vi "Teleop.vi"(1 "PreValue 2":bool, 3 "PreValue":bool, 9 "PreValue 3":bool, 10 "Match Info":T1={"Autonomous Elapsed Seconds"=0.0, "TeleOp Elapsed Seconds"=0.0, "Disabled Elapsed Seconds"=0.0, "Visited Autonomous"=FALSE, "Visited TeleOp"=FALSE, "Visited Disabled"=FALSE, "Autonomous Settings"={"Autonomous Style"=enum."Independent", "VI Refnum"=refnum}}, 11 "Call Context":T2) -> (0 "CurrentValue 2":bool, 2 "CurrentValue":bool, 8 "CurrentValue 3":bool)   [LabVIEW 2015]
doc: "This VI is called for each TeleOp packet received from the DS where the robot is not disabled. It is often used to read from the joysticks and update I/O or to update setpoints for timed control loops. It should complete and return within 20 milliseconds or it may miss DS packets."
uses:
  <vilib>/Rock Robotics/WPI/DriverStation/WPI_DriverStationDerivedRobotMode.ctl
  <vilib>/Rock Robotics/WPI/DriverStation/WPI_DriverStationMatch Info.ctl
  <vilib>/Rock Robotics/WPI/Solenoid/WPI_SolenoidValue.ctl
  <vilib>/Rock Robotics/WPI/Utilities/WPI_GetSetVariantRefNum.vi
  <vilib>/Rock Robotics/Network Tables/NT Write Boolean.vi
  <vilib>/Rock Robotics/Network Tables/NT Write Numeric Array.vi
  <vilib>/Rock Robotics/Network Tables/NT Read Boolean.vi
  <vilib>/Rock Robotics/Network Tables/NT Read Number.vi
  Robot Global Data.vi
  <vilib>/Rock Robotics/WPI/Solenoid/WPI_SolenoidSetEnum.vi
panel:
  out "Sample Slider 0":dbl(slide) scale=0.0..5.0
  out "Sample Boolean 1":bool
  out "Sample Boolean 0":bool
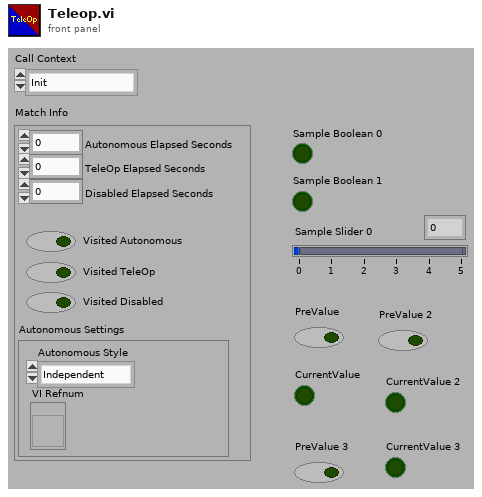
[diagram p1: front panel]
types:
  T1 = typedef "WPI_DriverStationMatch Info.ctl" = cluster{"Autonomous Elapsed Seconds":dbl, "TeleOp Elapsed Seconds":dbl, "Disabled Elapsed Seconds":dbl, "Visited Autonomous":bool, "Visited TeleOp":bool, "Visited Disabled":bool, "Autonomous Settings":cluster{"Autonomous Style":enum16{"Iterative", "Independent"}, "VI Refnum":refnum<vi>}}
  T2 = typedef "WPI_DriverStationDerivedRobotMode.ctl" = enum16{"Init", "Execute", "Stop"}
  T3 = typedef "WPI_RobotDriveDevRef.ctl" = cluster{"DevStatus":errorcluster, "Motors[]":T4[], "Square Inputs":bool, "Max Output":dbl}
  T4 = typedef "WPI_MotorControlDeviceRef.ctl" = cluster{"DeviceStatus":errorcluster, "Type":T5, "PWM":cluster{"PWM Channel":T6, "DeadBand":T7}, "CAN":cluster{"Device Number":u8, "Control Mode":T8, "Semaphore":T9, "Max Vout":dbl, "TalonSRX Control Mode":T10}, "Invert":bool}
  T5 = typedef "WPI_MotorControlType.ctl" = enum16{"PWM", "CAN", "CANTalonSRX"}
  T6 = typedef "FPGA_DIOPWMChannel.ctl" = enum8{"PWM 0", "PWM 1", "PWM 2", "PWM 3", "PWM 4", "PWM 5", "PWM 6", "PWM 7", "PWM 8", "PWM 9", "PWM MXP 0", "PWM MXP 1", "PWM MXP 2", "PWM MXP 3", "PWM MXP 4", "PWM MXP 5", "PWM MXP 6", "PWM MXP 7", "PWM MXP 8", "PWM MXP 9", "Invalid"}
  T7 = typedef "WPI_PWMDeadband.ctl" = cluster{"Name":string, "maxPositivePwm":i32, "minPositivePwm":i32, "centerPwm":i32, "maxNegativePwm":i32, "minNegativePwm":i32, "angularRange":u16}
  T8 = typedef "WPI_CANJaguar_ControlMode.ctl" = enum8{"Percent VBus", "Current", "Speed", "Position", "Voltage"}
  T9 = typedef "Semaphore RefNum" = refnum<k1>
  T10 = typedef "WPI_CANTalonSRX_APIControlMode.ctl" = enum8{"Percent VBus", "Speed", "Position", "Slave", "Unchanged / Invalid", "Voltage Compensation", "Current", "Motion Profile"}
  T11 = typedef "WPI_JoystickDevRef.ctl" = cluster{"Device":T12}
  T12 = typedef "WPI_JoystickDeviceEnum.ctl" = enum16{"USB 0", "USB 1", "USB 2", "USB 3", "USB 4", "USB 5"}
  T13 = cluster{"Buttons[0]":bool, "Buttons[1]":bool, "Buttons[2]":bool, "Buttons[3]":bool, "Buttons[4]":bool, "Buttons[5]":bool, "Buttons[6]":bool, "Buttons[7]":bool, "Buttons[8]":bool}
  T14 = typedef "WPI_DigitalInputDevRef.ctl" = cluster{"DevStatus":errorcluster, "DIO Channel":T15}
  T15 = typedef "FPGA_DIOChannel.ctl" = enum8{"DIO 0", "DIO 1", "DIO 2", "DIO 3", "DIO 4", "DIO 5", "DIO 6", "DIO 7", "DIO 8", "DIO 9", "DIO MXP 0", "DIO MXP 1", "DIO MXP 2", "DIO MXP 3", "DIO MXP 4", "DIO MXP 5", "DIO MXP 6", "DIO MXP 7", "DIO MXP 8", "DIO MXP 9", "DIO MXP 10", "DIO MXP 11", "DIO MXP 12", "DIO MXP 13", "DIO MXP 14", "DIO MXP 15", "Invalid"}
  T16 = typedef "WPI_SolenoidDevRef.ctl" = cluster{"DevStatus":errorcluster, "Pneumatics Control Module":u8, "Forward Solenoid Channel":T17, "Reverse Solenoid Channel":T17}
  T17 = typedef "WPI_SolenoidChannel.ctl" = enum8{"Solenoid 0", "Solenoid 1", "Solenoid 2", "Solenoid 3", "Solenoid 4", "Solenoid 5", "Solenoid 6", "Solenoid 7", "Invalid"}
  T18 = typedef "WPI_SolenoidValue.ctl" = enum16{"Off", "On", "Forward", "Reverse"}
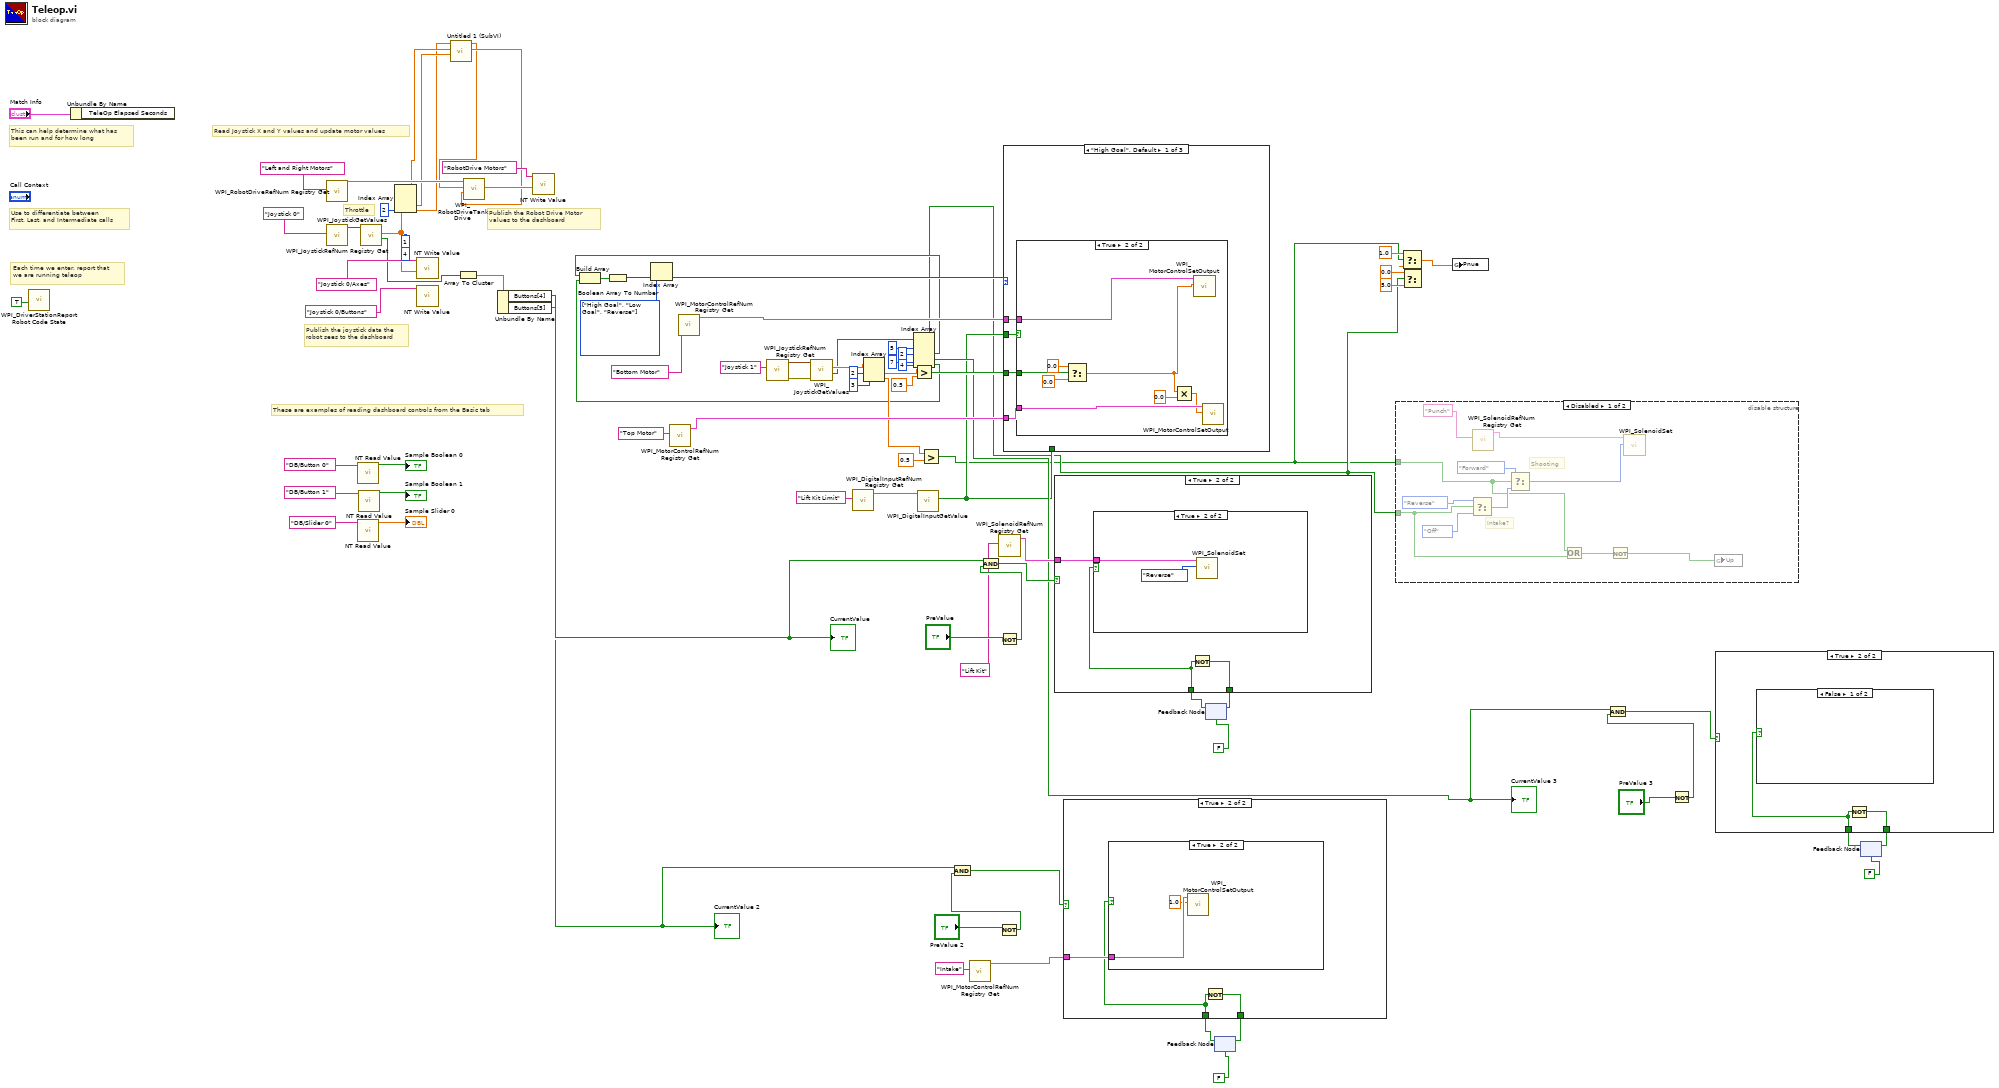
[diagram p0: block diagram]
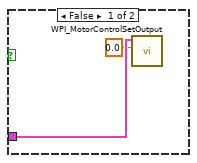
[diagram p6: hidden frame]
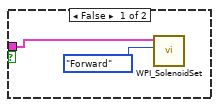
[diagram p8: hidden frame]
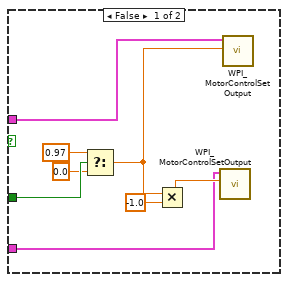
[diagram p9: hidden frame]
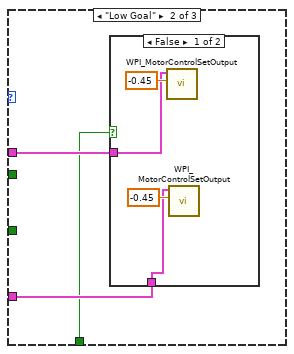
[diagram p10: hidden frame]
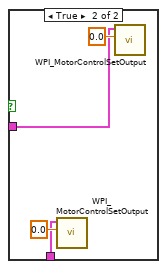
[diagram p11: hidden frame]
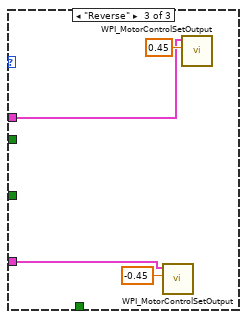
[diagram p12: hidden frame]
diagram:
  w70 = enum16{"High Goal", "Low Goal", "Reverse", ""}[] [enum."High Goal", enum."Low Goal", enum."Reverse"] items=["High Goal", "Low Goal", "Reverse", ""] ("array")
  # "Throttle"
  # "These are examples of reading dashboard controls from the Basic tab"
  # "Publish the Robot Drive Motor\nvalues to the dashboard"
  # "Publish the joystick data the\nrobot sees to the dashboard"
  # "Each time we enter, report that\nwe are running teleop"
  # "Use to differentiate between\nFirst, Last, and Intermediate calls"
  # "This can help determine what has\nbeen run and for how long"
  # "Read Joystick X and Y values and update motor values"
  n1 = call <vilib>:"WPI_DriverStationReport Robot Code State.vi"("TeleOp"=TRUE ("Autonomous")) -> ()  [unwired: 10 in, 1 out]
  n2 = Unbundle By Name("Match Info") -> ()  [unwired: 1 out]
  n3 = call <vilib>:"WPI_RobotDriveRefNum Registry Get.vi"("refnum name"="Left and Right Motors") -> ("RobotDriveDevRef"=w53:T3)  [unwired: 1 in, 9 out]
  n4 = call <vilib>:"WPI_JoystickRefNum Registry Get.vi"("refnum name"="Joystick 0") -> ("JoystickDevRef"=w85:T11)  [unwired: 1 in, 9 out]
  n5 = call-poly <vilib>:"NT Read Value.vi"("Name"="DB/Button 0" ("refnum name")) -> ("Boolean"=→"Sample Boolean 0":bool)  [unwired: 9 in, 1 out]
  n6 = call-poly <vilib>:"NT Read Value.vi"("Name"="DB/Slider 0" ("refnum name")) -> ("Numeric"=→"Sample Slider 0":dbl)  [unwired: 9 in, 1 out]
  n7 = call-poly <vilib>:"NT Read Value.vi"("Name"="DB/Button 1" ("refnum name")) -> ("Boolean"=→"Sample Boolean 1":bool)  [unwired: 9 in, 1 out]
  n8 = call <vilib>:"WPI_JoystickGetValues.vi"("JoystickDevRef"=w85) -> ("Buttons"=w66:bool[], "Axes"=w81:dbl[])  [unwired: 6 in, 3 out]
  n9 = Index Array(array=w81, index #1=1 ("index"), index #2=4 ("index"), index #3=2 ("index")) -> (element #1=w27:dbl, element #2=w28:dbl, element #3=w26:dbl)
  n10 = call-poly <vilib>:"NT Write Value.vi"("Numeric Array"=w81, "Name"="Joystick 0/Axes") -> ()  [unwired: 9 in, 1 out]
  n11 = call-poly <vilib>:"NT Write Value.vi"("Name"="Joystick 0/Buttons") -> ()  [unwired: 10 in, 1 out]
  n12 = call "Untitled 1 (SubVI).vi"("upper limit 2"=w28, "upper limit"=w27, "Throttle"=w26) -> ("Numeric 2"=w52:dbl, "Numeric"=w51:dbl)  [unwired: 7 in]
  n13 = Array To Cluster(array=w66) -> (cluster=w73:T13)
  n14 = call <vilib>:"WPI_RobotDriveTankDrive.vi"("Right axis value"=w52, "Left axis value"=w51, "RobotDriveDevRef"=w53) -> ("Motor Values"=w54:dbl[])  [unwired: 6 in, 2 out]
  n15 = Unbundle By Name(w73) -> ("Buttons[4]"=w63:bool, "Buttons[5]"=w31:bool)
  "CurrentValue" <- w63
  "CurrentValue 2" <- w31
  n16 = call-poly <vilib>:"NT Write Value.vi"("Numeric Array"=w54, "Name"="RobotDrive Motors") -> ()  [unwired: 9 in, 1 out]
  n17 = call <vilib>:"WPI_MotorControlRefNum Registry Get.vi"("refnum name"="Top Motor") -> ("MotorControlDevRef"=w64:T4)  [unwired: 9 in, 1 out]
  n18 = call <vilib>:"WPI_MotorControlRefNum Registry Get.vi"("refnum name"="Bottom Motor") -> ("MotorControlDevRef"=w68:T4)  [unwired: 9 in, 1 out]
  n19 = call <vilib>:"WPI_JoystickRefNum Registry Get.vi"("refnum name"="Joystick 1") -> ("error out"=w47:errorcluster, "JoystickDevRef"=w46:T11)  [unwired: 1 in, 8 out]
  n20 = call <vilib>:"WPI_JoystickGetValues.vi"("error in (no error)"=w47, "JoystickDevRef"=w46) -> ("Buttons"=w8:bool[], "Axes"=w44:dbl[])  [unwired: 5 in, 3 out]
  n21 = call <vilib>:"WPI_DigitalInputRefNum Registry Get.vi"("refnum name"="Lift Kit Limit") -> ("DigitalInputDevRef"=w11:T14)  [unwired: 9 in, 1 out]
  n22 = Index Array(array=w44, index #1=2 ("index"), index #2=3 ("index")) -> (element #1=w43:dbl, element #2=w38:dbl)
  n23 = Index Array(array=w8, index #1=5 ("index"), index #2=2 ("index"), index #3=7 ("index"), index #4=4 ("index")) -> (element #1=w2:bool, element #2=w14:bool, element #3=w20:bool, element #4=w12:bool)
  "CurrentValue 3" <- w20
  n24 = Build Array(w14, w12) -> (w72:bool[])
  n25 = Boolean Array To Number(Boolean array=w72) -> (number=w71:u32)
  n26 = Index Array(array=w70, index=w71) -> (element=w69:enum16{"High Goal", "Low Goal", "Reverse", ""})
  n27 = Greater?(x=w43, y=0.5) -> (0:w41:bool)
  n28 = call <vilib>:"WPI_DigitalInputGetValue.vi"("DigitalInputDevRef"=w11) -> ("Value"=w9:bool)  [unwired: 8 in, 2 out]
  n29 = Greater?(x=w38, y=0.5) -> (0:w1:bool)
  n30 = call <vilib>:"WPI_MotorControlRefNum Registry Get.vi"("refnum name"="Intake") -> ("MotorControlDevRef"=w33:T4)  [unwired: 9 in, 1 out]
  n31 = Not(x="PreValue 2") -> (.not. x?=w30:bool)
  n32 = And(x=w31, y=w30) -> (x .and. y?=w29:bool)
  n33 = call <vilib>:"WPI_SolenoidRefNum Registry Get.vi"("refnum name"="Lift Kit") -> ("SolenoidDevRef"=w55:T16)  [unwired: 9 in, 1 out]
  n34 = Not(x="PreValue") -> (.not. x?=w61:bool)
  n35 = And(x=w63, y=w61) -> (x .and. y?=w60:bool)
  n36 = case shown="\"High Goal\", Default" w69 {
    tunnel: w68 -> [w92 w111 w122]
    tunnel: w64 -> [w91 w110 w120]
    tunnel: w41 -> [w90 _ _]
    tunnel: w9 -> [_ w109 _]
    tunnel: w9 -> [w89 _ _]
    frame "High Goal", Default {
      n37 = case shown="True" w89 {
        tunnel: w92 -> [w94 w108]
        tunnel: w91 -> [w93 w107]
        tunnel: w90 -> [w99 w106]
        frame False {
          n38 = Select(t=0.97, s=w99, f=0.0) -> (s? t:f=w98:dbl)
          n39 = Multiply(x=w98, y=-1.0) -> (x*y=w100:dbl)
          n40 = call <vilib>:"WPI_MotorControlSetOutput.vi"("Output"=w100, "MotorControlDevRef"=w93) -> ()  [unwired: 7 in, 3 out]
          n41 = call <vilib>:"WPI_MotorControlSetOutput.vi"("Output"=w98, "MotorControlDevRef"=w94) -> ()  [unwired: 7 in, 3 out]
        }
        frame True {
          n42 = Select(t=0.0, s=w106, f=0.0) -> (s? t:f=w104:dbl)
          n43 = Multiply(x=w104, y=0.0) -> (x*y=w102:dbl)
          n44 = call <vilib>:"WPI_MotorControlSetOutput.vi"("Output"=w104, "MotorControlDevRef"=w108) -> ()  [unwired: 7 in, 3 out]
          n45 = call <vilib>:"WPI_MotorControlSetOutput.vi"("Output"=w102, "MotorControlDevRef"=w107) -> ()  [unwired: 7 in, 3 out]
        }
      }
    }
    frame "Low Goal" {
      n46 = case shown="False" w109 {
        tunnel: w111 -> [w112 w118]
        tunnel: w110 -> [w113 w116]
        frame False {
          n47 = call <vilib>:"WPI_MotorControlSetOutput.vi"("Output"=-0.45, "MotorControlDevRef"=w112) -> ()  [unwired: 7 in, 3 out]
          n48 = call <vilib>:"WPI_MotorControlSetOutput.vi"("Output"=-0.45, "MotorControlDevRef"=w113) -> ()  [unwired: 7 in, 3 out]
        }
        frame True {
          n49 = call <vilib>:"WPI_MotorControlSetOutput.vi"("Output"=0.0, "MotorControlDevRef"=w116) -> ()  [unwired: 7 in, 3 out]
          n50 = call <vilib>:"WPI_MotorControlSetOutput.vi"("Output"=0.0, "MotorControlDevRef"=w118) -> ()  [unwired: 7 in, 3 out]
        }
      }
    }
    frame "Reverse" {
      n51 = call <vilib>:"WPI_MotorControlSetOutput.vi"("Output"=-0.45, "MotorControlDevRef"=w120) -> ()  [unwired: 7 in, 3 out]
      n52 = call <vilib>:"WPI_MotorControlSetOutput.vi"("Output"=0.45, "MotorControlDevRef"=w122) -> ()  [unwired: 7 in, 3 out]
    }
  }
  n53 = feedback #1(FALSE) -> (w57:bool)
  n54 = case shown="True" w60 {
    tunnel: [w124 w127] -> w58
    tunnel: w57 -> [w124 w125]
    tunnel: w55 -> [_ w126]
    frame False {
    }
    frame True {
      n55 = case shown="True" w125 {
        tunnel: w126 -> [w129 w131]
        frame False {
          n56 = call-poly <vilib>:"WPI_SolenoidSet.vi"("Value"=WPI_SolenoidValue."Forward", "SolenoidDevRef"=w129) -> ()  [unwired: 8 in, 2 out]
        }
        frame True {
          n57 = call-poly <vilib>:"WPI_SolenoidSet.vi"("Value"=WPI_SolenoidValue."Reverse", "SolenoidDevRef"=w131) -> ()  [unwired: 8 in, 2 out]
        }
      }
      n58 = Not(x=w125) -> (.not. x?=w127:bool)
    }
  }
  n59 = feedback-in #1(w58) -> ()
  n60 = feedback #2(FALSE) -> (w34:bool)
  n61 = case shown="True" w29 {
    tunnel: [w132 w135] -> w35
    tunnel: w34 -> [w132 w133]
    tunnel: w33 -> [_ w134]
    frame False {
    }
    frame True {
      n62 = case shown="True" w133 {
        tunnel: w134 -> [w137 w139]
        frame False {
          n63 = call <vilib>:"WPI_MotorControlSetOutput.vi"("Output"=0.0, "MotorControlDevRef"=w137) -> ()  [unwired: 7 in, 3 out]
        }
        frame True {
          n64 = call <vilib>:"WPI_MotorControlSetOutput.vi"("Output"=1.0, "MotorControlDevRef"=w139) -> ()  [unwired: 7 in, 3 out]
        }
      }
      n65 = Not(x=w133) -> (.not. x?=w135:bool)
    }
  }
  n66 = feedback-in #2(w35) -> ()
  n67 = disable-structure shown="Disabled" {
    disable-tunnel: w1 -> [w143 _]
    disable-tunnel: w2 -> [w142 _]
    frame Disabled {
      # "Intake?"
      # "Shooting"
      n68 = Select(t=WPI_SolenoidValue."Reverse" ("Value"), s=w142, f=WPI_SolenoidValue."Off" ("Value")) -> (s? t:f=w146:T18)
      n69 = call <vilib>:"WPI_SolenoidRefNum Registry Get.vi"("refnum name"="Punch") -> ("SolenoidDevRef"=w150:T16)  [unwired: 9 in, 1 out]
      n70 = Select(t=WPI_SolenoidValue."Forward" ("Value"), s=w143, f=w146) -> (s? t:f=w149:T18)
      n71 = Or(x=w143, y=w142) -> (x .or. y?=w141:bool)
      n72 = Not(x=w141) -> (.not. x?=w140:bool)
      n73 = call-poly <vilib>:"WPI_SolenoidSet.vi"("Value"=w149, "SolenoidDevRef"=w150) -> ()  [unwired: 8 in, 2 out]
      n74 = global write "Robot Global Data.vi" "Up"(w140) -> ()
    }
    frame Enabled {
    }
  }
  n75 = Select(t=0.0, s=w2, f=5.0) -> (s? t:f=w4:dbl)
  n76 = Select(t=1.0, s=w1, f=w4) -> (s? t:f=w3:dbl)
  n77 = global write "Robot Global Data.vi" "Pnue"(w3) -> ()
  n78 = Not(x="PreValue 3") -> (.not. x?=w21:bool)
  n79 = And(x=w20, y=w21) -> (x .and. y?=w19:bool)
  n80 = feedback #3(FALSE) -> (w16:bool)
  n81 = case shown="True" w19 {
    tunnel: [w151 w153] -> w17
    tunnel: w16 -> [w151 w152]
    frame False {
    }
    frame True {
      n82 = case shown="False" w152 {
        frame False {
        }
        frame True {
        }
      }
      n83 = Not(x=w152) -> (.not. x?=w153:bool)
    }
  }
  n84 = feedback-in #3(w17) -> ()
